vi "www template error.vi"(6 "User Information":T1, 8 "error in (no error)":errorcluster, 11 "Incoming Template HTML (\"\")":string) -> (3 "error.htm":string)   [LabVIEW 2011]
uses:
  server/database/Users/User Record.ctl
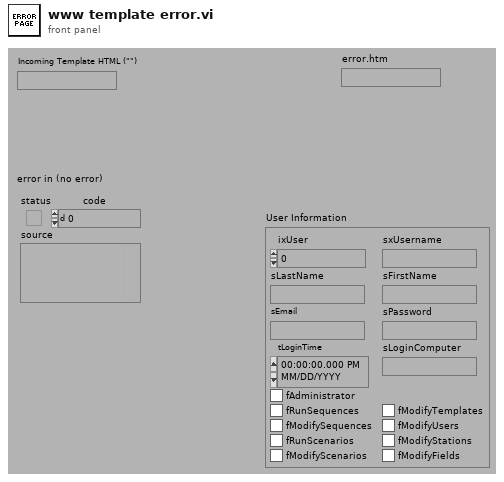
[diagram p1: front panel]
types:
  T1 = typedef "User Record.ctl" = cluster{"ixUser":i32, "sxUsername":string, "sLastName":string, "sFirstName":string, "sEmail":string, "sPassword":string, "tLoginTime":timestamp, "sLoginComputer":string, "fAdministrator":bool, "fRunSequences":bool, "fModifySequences":bool, "fRunScenarios":bool, "fModifyScenarios":bool, "fModifyTemplates":bool, "fModifyUsers":bool, "fModifyStations":bool, "fModifyFields":bool}
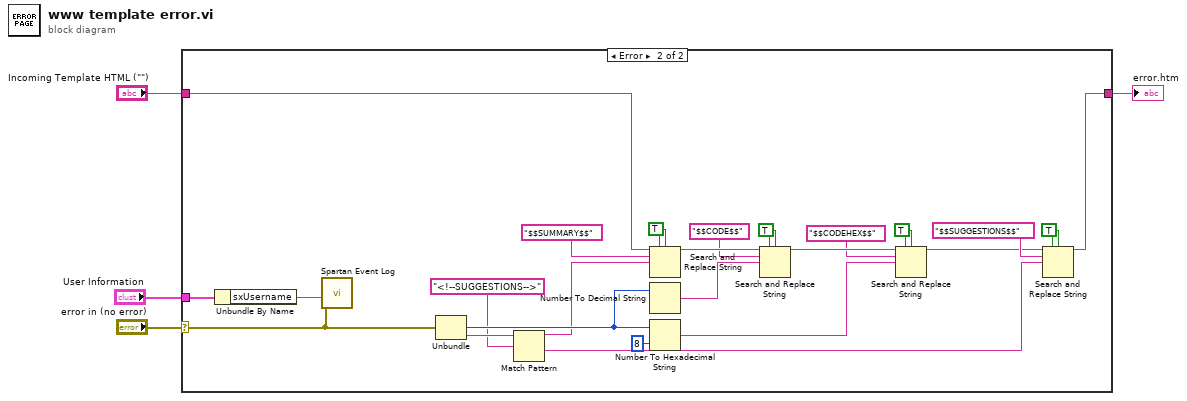
[diagram p0: block diagram]
diagram:
  n1 = case shown="Error" "error in (no error)" {
    selector: "error in (no error)" -> [_ w8]
    tunnel: [w5 w14] -> w4
    tunnel: "Incoming Template HTML (\"\")" -> [w5 w9]
    tunnel: "User Information" -> [_ w7]
    frame No Error {
    }
    frame Error {
      w16 = TRUE
      w23 = TRUE
      w26 = TRUE
      w28 = TRUE
      n2 = Unbundle By Name(w7) -> ("sxUsername"=w6:string)
      n3 = call "Spartan Event Log.vi"("error in (no error)"=w8, "username (\"\")"=w6) -> ()  [unwired: 6 in, 1 out]
      n4 = Unbundle(w8) -> ("code"=w19:i32, "source"=w13:string)  [unwired: 1 out]
      n5 = Match Pattern(string=w13, regular expression="<!--SUGGESTIONS-->") -> (before substring=w12:string, after substring=w10:string)  [unwired: 3 out]
      n6 = Search and Replace String(replace all?=w28, case sensitive?=w28, input string=w9, search string="$$SUMMARY$$", replace string=w12) -> (result string=w25:string)  [unwired: 1 in, 5 out]
      n7 = Number To Decimal String(number=w19) -> (decimal integer string=w18:string)  [unwired: 1 out]
      n8 = Number To Hexadecimal String(1:i16 8 ("width (-)"), 2:w19) -> (0:w20:string)
      n9 = Search and Replace String(replace all?=w26, case sensitive?=w26, input string=w25, search string="$$CODE$$", replace string=w18) -> (result string=w22:string)  [unwired: 1 in, 5 out]
      n10 = Search and Replace String(replace all?=w23, case sensitive?=w23, input string=w22, search string="$$CODEHEX$$", replace string=w20) -> (result string=w15:string)  [unwired: 1 in, 5 out]
      n11 = Search and Replace String(replace all?=w16, case sensitive?=w16, input string=w15, search string="$$SUGGESTIONS$$", replace string=w10) -> (result string=w14:string)  [unwired: 1 in, 5 out]
    }
  }
  "error.htm" <- w4
